vi "CfgFile Read Configuration File.vi"(8 "error in (no error)":errorcluster, 11 "LF2R IDE in":refnum<class "Main Panel.lvclass">) -> (0 "error out":errorcluster, 1 "Exist?":bool, 2 "Config Data":T1={"Language"={"Name"=""}, "Path Config"={"Data Folder Path"=path "", "PNG Folder Path"=path ""}, "Image Viewer Config"={"Center Point"={"Size"=3, "Color"=0, "Show?"=FALSE}, "bp Point"={"Size"=3, "Color"=0, "Show?"=FALSE}, "w Point"={"Size"=3, "Color"=0, "Show?"=FALSE}, "b Box"={"Fill Color"=0, "Border Color"=0, "Show?"=FALSE}, "i Box"={"Fill Color"=0, "Border Color"=0, "Show?"=FALSE}, "o Point"={"Size"=3, "Color"=0, "Show?"=FALSE}, "c Point"={"Size"=3, "Color"=0, "Show?"=FALSE}}}, 3 "LF2R IDE out":refnum<class "Main Panel.lvclass">)   [LabVIEW 2018, in "Main Panel.lvlib" / "Main Panel.lvclass"]
uses:
  Main Panel.lvclass
  Const Configuration.ctl
  Const Path Setting.ctl
  Const Image Viewer Setting.ctl
  136ff03b-022a-4f22-8316-e9f628dcce0b.vi
  <vilib>/JDP Science/JSONtext/JSON text to Variant.vi
  <vilib>/JDP Science/JSONtext/LVClass Serializer/JSONtext LVClass Serializer.lvclass
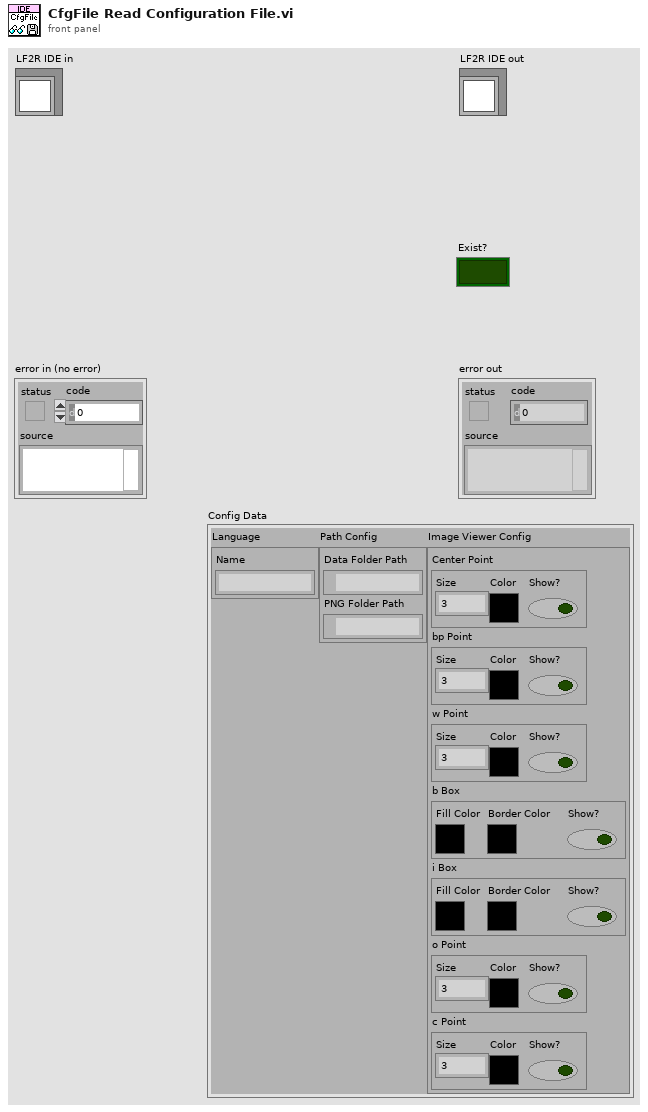
[diagram p1: front panel]
types:
  T1 = typedef "Main Panel.lvlib/Main Panel.lvclass/Const Configuration.ctl" = cluster{"Language":cluster{"Name":string}, "Path Config":T2, "Image Viewer Config":T3}
  T2 = typedef "Main Panel.lvlib/Main Panel.lvclass/Const Path Setting.ctl" = cluster{"Data Folder Path":path, "PNG Folder Path":path}
  T3 = typedef "Main Panel.lvlib/Main Panel.lvclass/Const Image Viewer Setting.ctl" = cluster{"Center Point":cluster{"Size":i32, "Color":u32, "Show?":bool}, "bp Point":cluster{"Size":i32, "Color":u32, "Show?":bool}, "w Point":cluster{"Size":i32, "Color":u32, "Show?":bool}, "b Box":cluster{"Fill Color":u32, "Border Color":u32, "Show?":bool}, "i Box":cluster{"Fill Color":u32, "Border Color":u32, "Show?":bool}, "o Point":cluster{"Size":i32, "Color":u32, "Show?":bool}, "c Point":cluster{"Size":i32, "Color":u32, "Show?":bool}}
  T4 = enum16{"open", "replace", "create", "open or create", "replace or create", "replace or create with confirmation"}
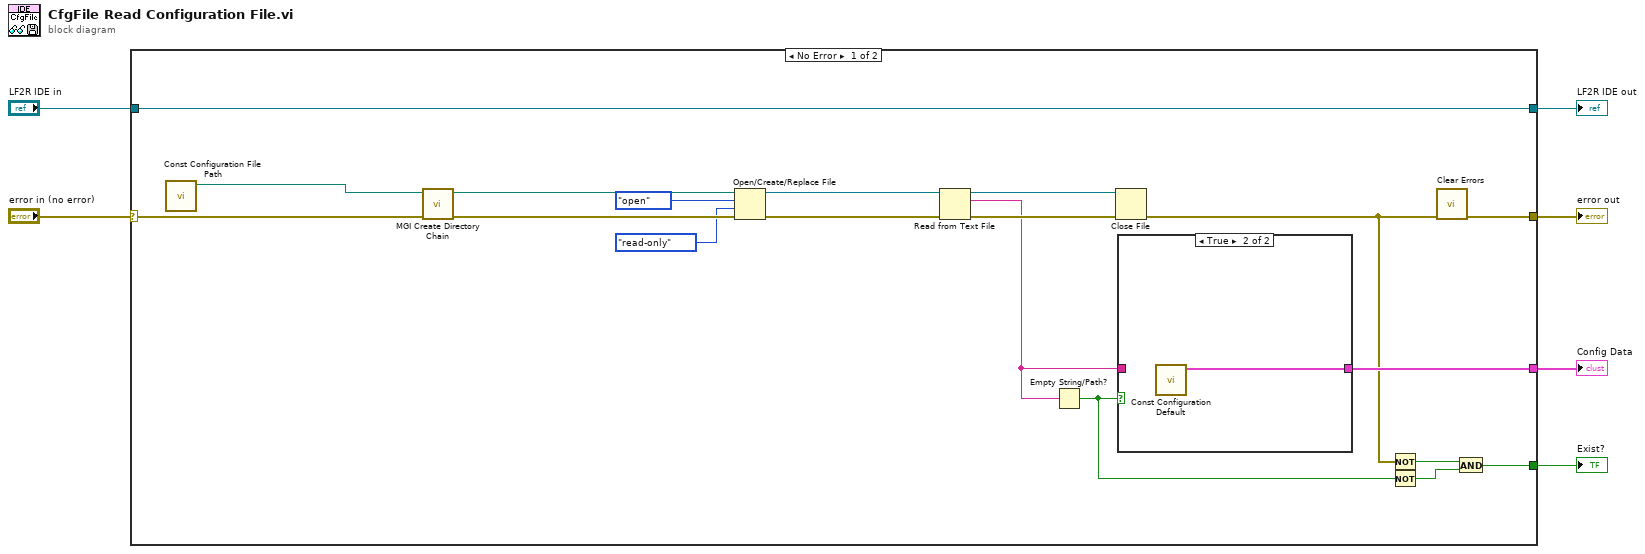
[diagram p0: block diagram]
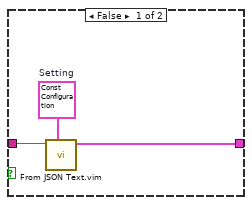
[diagram p2: hidden frame]
diagram:
  n1 = case shown="No Error" "error in (no error)" {
    selector: "error in (no error)" -> [w17 w31]
    tunnel: [w12 w31] -> w5
    tunnel: [w18 w30] -> w3
    tunnel: "LF2R IDE in" -> [w18 w30]
    tunnel: [w13 _] -> w2
    tunnel: [w9 _] -> w1
    frame No Error {
      n2 = call "Const Configuration File Path.vi"() -> ("Config File Path"=w20:path)  [unwired: 11 in]
      n3 = call <userlib>:"MGI Create Directory Chain.vi"("Error In"=w17, "Path"=w20) -> ("Error Out"=w24:errorcluster, "Duplicate Path"=w25:path)  [unwired: 8 in]
      n4 = Open/Create/Replace File(file path (use dialog)=w25, error in=w24, operation (0:open)=T4."open", access (0:read/write)=enum16{"read/write", "read-only", "write-only"}."read-only") -> (refnum out=w23:refnum<file>, error out=w22:errorcluster)  [unwired: 2 in, 1 out]
      n5 = Read from Text File(file (use dialog)=w23, error in=w22) -> (refnum out=w21:refnum<file>, text=w14:string, error out=w16:errorcluster)  [unwired: 2 in, 1 out]
      n6 = Empty String/Path?(string/path=w14) -> (empty?=w11:bool)
      n7 = Close File(refnum=w21, error in=w16) -> (error out=w7:errorcluster)  [unwired: 1 out]
      n8 = case shown="True" w11 {
        tunnel: [w26 w29] -> w13
        tunnel: w14 -> [w27 _]
        frame False {
          w28 = T1 {"Language"={"Name"=""}, "Path Config"={"Data Folder Path"=path "", "PNG Folder Path"=path ""}, "Image Viewer Config"={"Center Point"={"Size"=3, "Color"=0, "Show?"=FALSE}, "bp Point"={"Size"=3, "Color"=0, "Show?"=FALSE}, "w Point"={"Size"=3, "Color"=0, "Show?"=FALSE}, "b Box"={"Fill Color"=0, "Border Color"=0, "Show?"=FALSE}, "i Box"={"Fill Color"=0, "Border Color"=0, "Show?"=FALSE}, "o Point"={"Size"=3, "Color"=0, "Show?"=FALSE}, "c Point"={"Size"=3, "Color"=0, "Show?"=FALSE}}}  # Setting
          n9 = call "From JSON Text.vim"("Data Type and Default Value"=w28, "JSON"=w27) -> ("Data out"=w26:T1)  [unwired: 8 in, 1 out]
        }
        frame True {
          n10 = call "Const Configuration Default.vi"() -> ("Config"=w29:T1)  [unwired: 11 in]
        }
      }
      n11 = Not(x=w7) -> (.not. x?=w10:bool)
      n12 = Not(x=w11) -> (.not. x?=w8:bool)
      n13 = call <vilib>:"Clear Errors.vi"("error in (no error)"=w7) -> ("error out"=w12:errorcluster)  [unwired: 5 in, 1 out]
      n14 = And(x=w10, y=w8) -> (x .and. y?=w9:bool)
    }
    frame Error {
    }
  }
  "error out" <- w5
  "LF2R IDE out" <- w3
  "Config Data" <- w2
  "Exist?" <- w1
